vi "State Enqueue.vi"(8 "error in (no error)":errorcluster, 9 "Display State Change Class":T1, 11 "Control Ref Queue":T2) -> (0 "error out":errorcluster)   [LabVIEW 2020, in "2D Plot.lvclass"]
uses:
  <vilib>/Math Plots/2D Math Plots/2D Plot/2D Plot/2D Plot.lvclass
  <vilib>/Math Plots/2D Math Plots/2D Plot/Action String/2DMathPlot Ctrl Act Queue.ctl
  <vilib>/Math Plots/2D Math Plots/2D Plot/Action String/2DMathPlot Ctrl Act Cluster.ctl
  <vilib>/Math Plots/2D Math Plots/2D Plot/Action String/2DMathPlot State Class.ctl
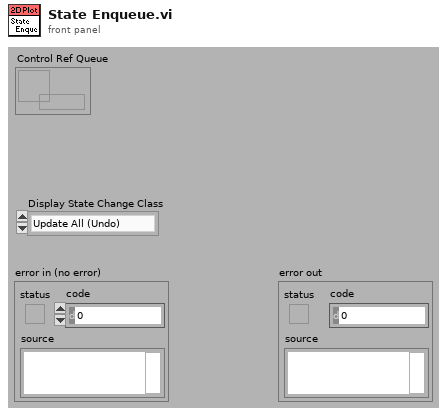
[diagram p1: front panel]
types:
  T1 = typedef "2DMathPlot State Class.ctl" = enum16{"Update All (Undo)", "Update General", "Update Appearance", "Update Format", "Update Scale", "Update Marker", "Update Cursor", "None"}
  T2 = typedef "2DMathPlot Ctrl Act Queue.ctl" = refnum<queue>
  T3 = typedef "2DMathPlot Ctrl Act Cluster.ctl" = cluster{"Plot Area Ref":refnum<vi>, "Z Axis Ref":refnum<vi>, "Legend Ref":refnum<vi>, "XControl Ref":refnum<vi>, "Facade Ref":refnum<vi>, "Display State Change Class":T1}
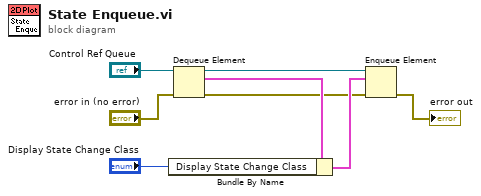
[diagram p0: block diagram]
diagram:
  n1 = Dequeue Element(queue="Control Ref Queue", error in (no error)="error in (no error)") -> (queue out=w8:T2, element=w7:T3, error out=w5:errorcluster)  [unwired: 2 out]
  n2 = Bundle By Name(cluster=w7, "Display State Change Class"="Display State Change Class") -> (w6:T3)
  n3 = Enqueue Element(queue=w8, element=w6, error in (no error)=w5) -> (error out=→"error out":errorcluster)  [unwired: 3 out]
